vi "ramp.vi"(11 "Coagulant":T1={"flocculator volume (L)"=100.0, "clarifier volume (L)"=0.0, "dose updates per HRT"=0, "target clarified turbidity (NTU)"=0.3, "Coagulant mode"=enum."manual", "Coag dose [mg/L]"=0.0, "pump mL/rev"=0.0, "clarifier flow [L/s]"=0.5, "min Coag dose [mg/L]"=0.0, "max Coag dose [mg/L]"=0.0, "Steps"=3, "HRT response delay"=1, "Ku*"=1.0} {"HRT response delay" min=1 max=10 step=1; "Steps" min=3 step=1; "clarifier flow [L/s]" min=0.0001 max=1.0 step=0.0001; "target clarified turbidity (NTU)" min=0.1 max=5.0 step=0.01; "dose updates per HRT" min=1 max=100 step=1}) -> (3 "Coag dose":dbl)   [LabVIEW 2015]
uses:
  model type.ctl
  coag.ctl
panel:
  out "Numeric":i64
  # "min"
  # "max"
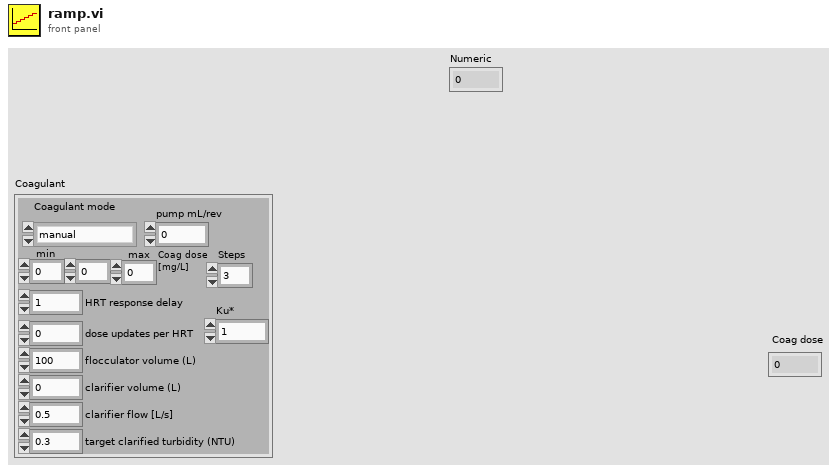
[diagram p1: front panel]
types:
  T1 = typedef "coag.ctl" = cluster{"flocculator volume (L)":dbl, "clarifier volume (L)":dbl, "dose updates per HRT":u16, "target clarified turbidity (NTU)":dbl, "Coagulant mode":T2, "Coag dose [mg/L]":dbl, "pump mL/rev":dbl, "clarifier flow [L/s]":dbl, "min Coag dose [mg/L]":dbl, "max Coag dose [mg/L]":dbl, "Steps":u16, "HRT response delay":u32, "Ku*":dbl}
  T2 = typedef "model type.ctl" = enum16{"manual", "ramp", "simple corrector", "linear regression"}
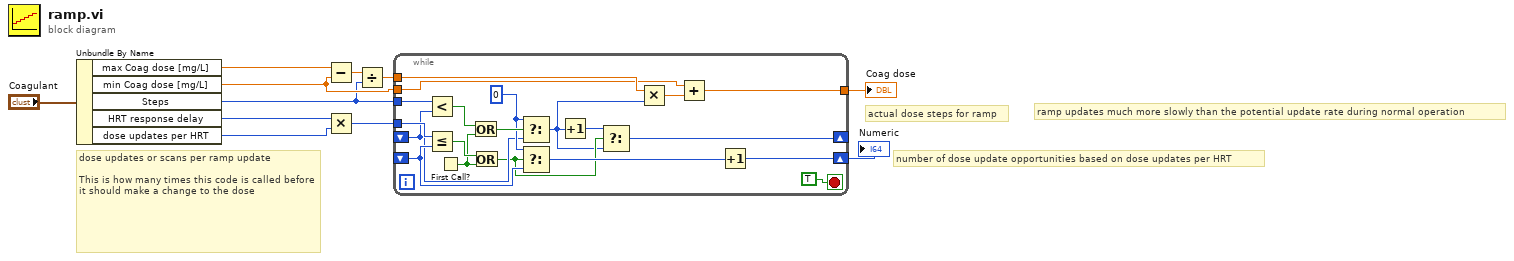
[diagram p0: block diagram]
diagram:
  # "ramp updates much more slowly than the potential update rate during normal operation"
  # "actual dose steps for ramp"
  # "number of dose update opportunities based on dose updates per HRT"
  # "dose updates or scans per ramp update\n\nThis is how many times this code is called before it should make a change to the dose"
  n1 = Unbundle By Name("Coagulant") -> ("max Coag dose [mg/L]"=w7:dbl, "min Coag dose [mg/L]"=w10:dbl, "Steps"=w1:u16, "HRT response delay"=w5:u32, "dose updates per HRT"=w4:u16)
  n2 = Subtract(x=w7, y=w10) -> (x-y=w9:dbl)
  n3 = Multiply(x=w5, y=w4) -> (x*y=w3:u32)
  n4 = Divide(x=w9, y=w1) -> (x/y=w8:dbl)
  n5 = while {
    tunnel: w10 -> [w26]
    tunnel: w8 -> [w28]
    shift-right: [w14] -> _
    shift-left: _ -> [w16]
    tunnel: w3 -> [w30]
    tunnel: [w25] -> w6
    shift-right: [w23] -> w2
    shift-left: _ -> [w22]
    tunnel: w1 -> [w21]
    stop <- TRUE stop-if-true
    w17 = i64 0 ("t")
    n6 = Less?(x=w21, y=w16) -> (x < y?=w20:bool)
    n7 = Less Or Equal?(x=w30, y=w22) -> (x <= y?=w29:bool)
    n8 = First Call?() -> (First Call?: T/F=w19:bool)
    n9 = Or(x=w20, y=w19) -> (x .or. y?=w18:bool)
    n10 = Or(x=w29, y=w19) -> (x .or. y?=w13:bool)
    n11 = Select(t=w17, s=w18, f=w16) -> (s? t:f=w12:i64)
    n12 = Select(t=w17, s=w13, f=w22) -> (s? t:f=w24:i64)
    n13 = Increment(x=w12) -> (x+1=w15:i64)
    n14 = Select(t=w15, s=w13, f=w12) -> (s? t:f=w14:i64)
    n15 = Multiply(x=w28, y=w12) -> (x*y=w27:dbl)
    n16 = Add(x=w26, y=w27) -> (x+y=w25:dbl)
    n17 = Increment(x=w24) -> (x+1=w23:i64)
  }
  "Coag dose" <- w6
  "Numeric" <- w2
